vi "ParseCommands.vi"(0 "ArrayType":string[](array[string]), 1 "Priority? (f)":bool, 5 "Script In":string[](array[string]), 7 "Delimiter (Tab)":string=",", 9 "Format string":string="%s", 11 "ErrorArrayIn":errorcluster[](array[cluster])) -> (4 "States":string[][](array[string]), 15 "ErrorArrayOut":errorcluster[](array[cluster]))   [LabVIEW 2018, in "Test.lvclass"]
doc: "Parses the commands in the SpreadSheetString and enqueus the script state as well as any data needed for the state to execute appropriately. This VI assumes that the state is the first value in the string entry seperated by a comma, example State, statedata."
uses:
  Test.lvclass
panel:
  out "Parameters":string[][](array[string])
  out "Commands":string[](array[string])
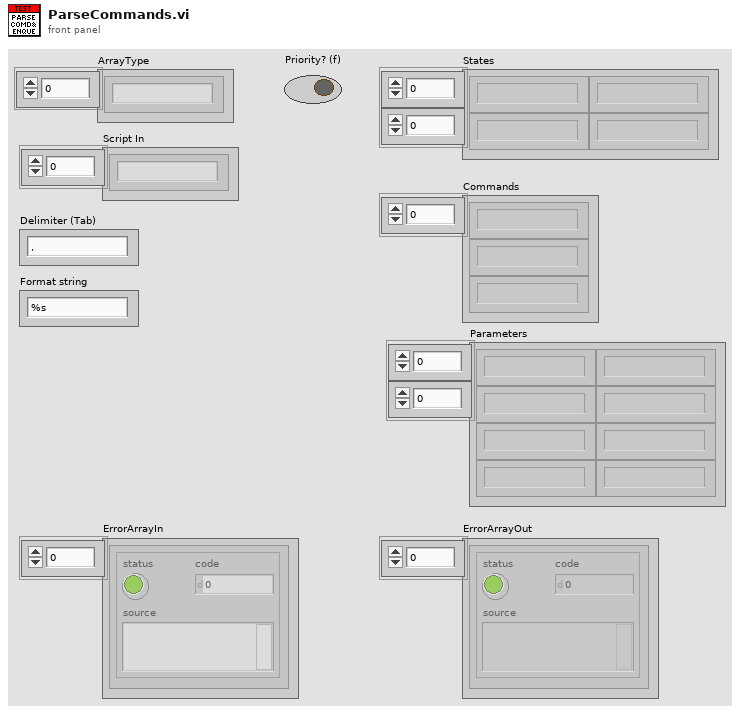
[diagram p1: front panel]
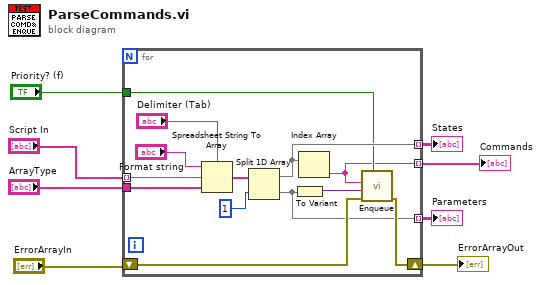
[diagram p0: block diagram]
diagram:
  n1 = for {
    tunnel: "Script In" -> [w19] mode=indexing
    shift-right: [w13] -> w5
    shift-left: "ErrorArrayIn" -> [w14]
    tunnel: "ArrayType" -> [w18]
    tunnel: [w12] -> w4 mode=indexing
    tunnel: "Priority? (f)" -> [w11]
    tunnel: [w10] -> w2 mode=indexing
    tunnel: [w9] -> w1 mode=indexing
    n2 = Spreadsheet String To Array(delimiter (Tab)="Delimiter (Tab)", format string="Format string", spreadsheet string=w19, array type (2D Dbl)=w18) -> (array=w16:string[])
    n3 = Split 1D Array(array=w16, index=1) -> (first subarray=w12:string[], second subarray=w9:string[])
    n4 = To Variant(anything=w9) -> (Variant=w15:variant)
    n5 = Index Array(array=w12) -> (element=w10:string)  [unwired: 1 in]
    n6 = call "Enqueue.vi"("Priority? (f)"=w11, "ErrorArray"=w14, "Data"=w15, "Message"=w10) -> ("ErrorArray"=w13:errorcluster[])  [unwired: 7 in]
  }
  "ErrorArrayOut" <- w5
  "States" <- w4
  "Commands" <- w2
  "Parameters" <- w1
